vi "Get Serials of All Controllers (uSMC).vi"(8 "error in (no error)":errorcluster, 10 "axis":i32, 11 "Visa array in":refnum<visa-resource-name>[](array[refnum])) -> (0 "error out":errorcluster, 2 "Serials":string, 3 "Visa array out":refnum<visa-resource-name>[](array[refnum]))   [LabVIEW 2010, in "SignalWriterMH110203USBStepperMotor.lvclass"]
uses:
  SignalWriterMH110203USBStepperMotor.lvclass
  class_data.vi
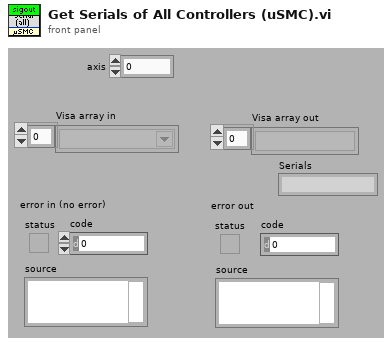
[diagram p1: front panel]
types:
  T1 = typedef "SignalWriterMH110203USBStepperMotor.lvclass/GoTo Control (uSMC).ctl" = cluster{"Step motor ID":string, "SMname":string, "Backlash":u16, "wait for input sygnal to start":bool, "use slow start/stop":bool, "units name":string, "Maximum speed":dbl, "speed":dbl, "step":u8, "point 1 ticks":i32, "point 2 ticks":i32, "point 1 units":dbl, "point 2 units":dbl, "Limit Switch standoff":dbl, "Zero Value":dbl, "Destination Position":dbl, "force backlash":bool, "power off when stop":bool, "POff delay":dbl, "positioner name":string, "R, Ohm":dbl, "I, mA":dbl, "Positioner's Type":u16, "Reset Direction":bool, "Manufacturer":string, "Model":string, "Scheme":string, "FirmwareVer":string}
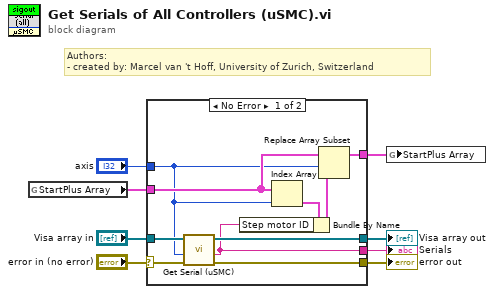
[diagram p0: block diagram]
diagram:
  # "Authors: \n- created by: Marcel van 't Hoff, University of Zurich, Switzerland"
  n1 = global read "class_data.vi" "StartPlus Array"() -> (w5:T1[])
  n2 = case shown="No Error" "error in (no error)" {
    selector: "error in (no error)" -> [w14 w21]
    tunnel: "Visa array in" -> [w18 w20]
    tunnel: [w17 w20] -> w7
    tunnel: [w16 w21] -> w6
    tunnel: w5 -> [w12 w19]
    tunnel: [w10 w19] -> w4
    tunnel: [w15 _] -> w3
    tunnel: "axis" -> [w9 _]
    frame No Error {
      n3 = call "Get Serial (uSMC).vi"("error in (no error)"=w14, "Index"=w9, "Visa array in"=w18) -> ("error out"=w16:errorcluster, "Serial Number"=w15:string, "Visa array out"=w17:refnum<visa-resource-name>[])  [unwired: 6 in]
      n4 = Index Array(array=w12, index=w9) -> (element=w13:T1)
      n5 = Bundle By Name(cluster=w13, "Step motor ID"=w15) -> (w11:T1)
      n6 = Replace Array Subset(array=w12, new element=w11, index=w9) -> (w10:T1[])
    }
    frame Error {
    }
  }
  "Visa array out" <- w7
  "error out" <- w6
  "Serials" <- w3
  n7 = global write "class_data.vi" "StartPlus Array"(w4) -> ()
